vi "Convert Time to String.vi"(10 "time stamp":timestamp, 11 "time format string (%c)":string="%Y-%m-%d %H:%M:%S") -> (3 "date/time string":string)   [LabVIEW 2014]
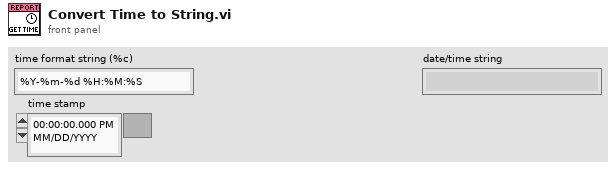
[diagram p1: front panel]
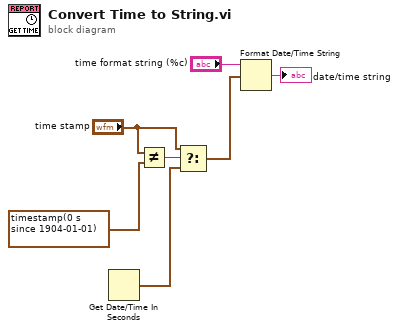
[diagram p0: block diagram]
diagram:
  n1 = Get Date/Time In Seconds() -> (seconds since 1Jan1904=w4:timestamp)
  n2 = Not Equal?(x="time stamp", y=timestamp(0 s since 1904-01-01) ("time stamp")) -> (x != y?=w5:bool)
  n3 = Select(t="time stamp", s=w5, f=w4) -> (s? t:f=w2:timestamp)
  n4 = Format Date/Time String(time format string (%c)="time format string (%c)", seconds (now)=w2) -> (date/time string=→"date/time string":string)  [unwired: 1 in]
